vi "cm2nm_save_sample_information.vi"(1 "Sample_Information":T1, 2 "Sample_data_base":path) -> (0 "Sample_data_base 2":path)   [LabVIEW 2011]
doc: "Save the main data base file for a sample into the XML file format and replace the old file."
uses:
  <vilib>/Utility/xml.llb/Write to XML File(string).vi
panel:
  out "error out":errorcluster
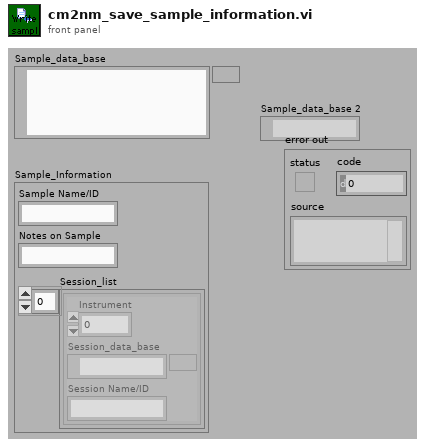
[diagram p1: front panel]
types:
  T1 = cluster{"Sample Name/ID":string, "Notes on Sample":string, "Session_list":cluster{"Instrument":u16, "Session_data_base":path, "Session Name/ID":string}[]}
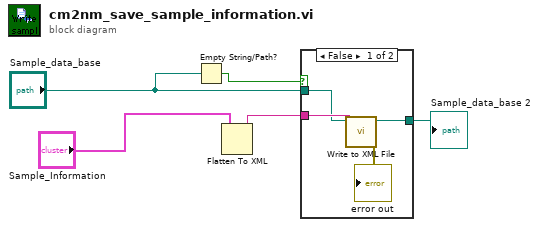
[diagram p0: block diagram]
diagram:
  n1 = Empty String/Path?(string/path="Sample_data_base") -> (empty?=w5:bool)
  n2 = Flatten To XML(anything="Sample_Information") -> (xml string=w1:string)
  n3 = case shown="False" w5 {
    tunnel: w1 -> [w9 _]
    tunnel: [w8 w10] -> w3
    tunnel: "Sample_data_base" -> [w7 w10]
    frame False {
      n4 = call-poly <vilib>:"Write to XML File.vi"("XML Input"=w9, "XML File Path"=w7) -> ("error out"=→"error out":errorcluster, "XML File Path(duplicate)"=w8:path)  [unwired: 3 in, 5 out]
    }
    frame True {
    }
  }
  "Sample_data_base 2" <- w3
